vi "Refname to String all.vi"   [LabVIEW 2016]
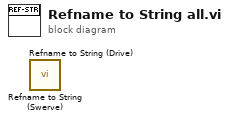
[diagram p0: block diagram]
diagram:
  n1 = call "Refname to String (Swerve).vi"() -> ()  [unwired: 5 in, 1 out]
  n2 = call "Refname to String (Drive).vi"() -> ()  [unwired: 5 in, 1 out]
